vi "Test Method Not Dashed.vi"(8 "error in (no error)":errorcluster, 11 "Dummy Test Case in":refnum<class "Dummy With Dashed Method.lvclass">) -> (0 "error out":errorcluster, 3 "Dummy Test Case out":refnum<class "Dummy With Dashed Method.lvclass">)   [LabVIEW 2020, in "Dummy With Dashed Method.lvclass"]
uses:
  Dummy With Dashed Method.lvclass
  C:/git/astemes-lunit/source/API/LUnit Test Case/LUnit Test Case.lvclass
  source/API/LUnit Test Case/LUnit Test Case.lvclass/LUnit Test Case.ctl
  source/API/LUnit Test Case/Private/Append Fail Result.vi
  Dummy With Dashed Method.lvclass/Dummy With Dashed Method.ctl
  source/API/LUnit Test Case/LUnit Test Case.lvclass
  C:/git/astemes-lunit/source/Core/Runnable/Runnable.lvclass
  C:/git/astemes-lunit/tests/Filter Test/Dummy With Dashed Method/Dummy With Dashed Method.lvclass
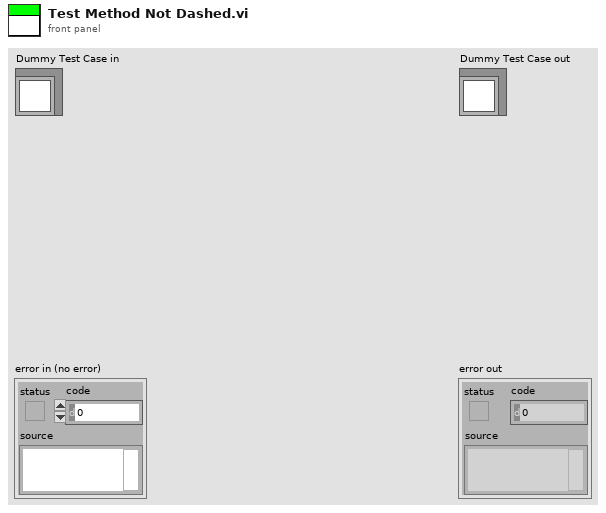
[diagram p1: front panel]
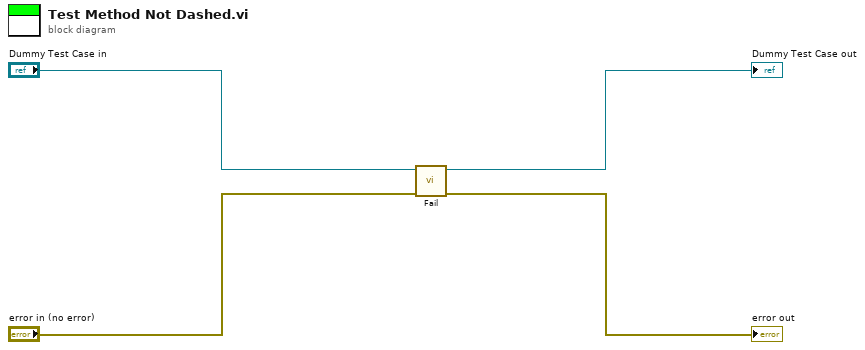
[diagram p0: block diagram]
diagram:
  n1 = call "Fail.vi"("error in (no error)"="error in (no error)", "LUnit Test Case In"="Dummy Test Case in") -> ("error out"=→"error out":errorcluster, "LUnit Test Case Out"=→"Dummy Test Case out":refnum<class "Dummy With Dashed Method.lvclass">)  [unwired: 8 in]
